vi "LVClasse_SurfaceFloat Read SurfaceFloat.vi"(8 "error in (no error)":errorcluster, 11 "SurfaceFloat in":refnum<class "SurfaceFloat.lvclass">) -> (0 "error out":errorcluster, 2 "SurfaceFloat":T1, 3 "SurfaceFloat out":refnum<class "SurfaceFloat.lvclass">)   [LabVIEW 2020, in "SurfaceFloat.lvclass"]
uses:
  SurfaceFloat.lvclass
  ClassID.ctl
  SurfaceFloat.lvclass/SurfaceFloat.ctl
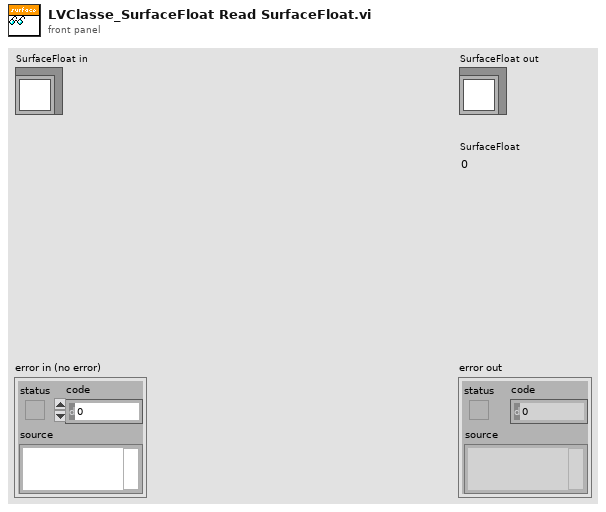
[diagram p1: front panel]
types:
  T1 = typedef "ClassID.ctl" = i64
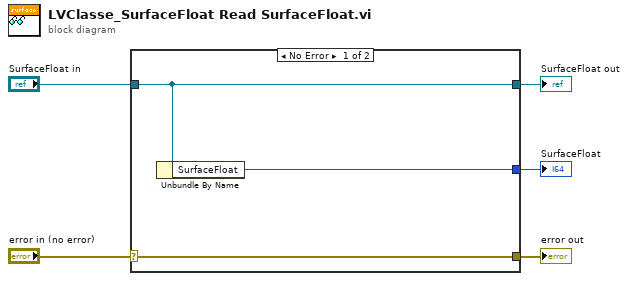
[diagram p0: block diagram]
diagram:
  n1 = case shown="No Error" "error in (no error)" {
    selector: "error in (no error)" -> [w8 w9]
    tunnel: [w8 w9] -> w4
    tunnel: [w7 w10] -> w2
    tunnel: "SurfaceFloat in" -> [w7 w10]
    tunnel: [w6 _] -> w1
    frame No Error {
      n2 = Unbundle By Name(w7) -> ("SurfaceFloat"=w6:T1)
    }
    frame Error {
    }
  }
  "error out" <- w4
  "SurfaceFloat out" <- w2
  "SurfaceFloat" <- w1
